vi "set_PSG.vi"(4 "PSG1 frequency":dbl) -> ()   [LabVIEW 2011]
doc: "sets PSG1 and PSG2 frequencies based on the frequency wired to the vi and the frequency offset stored in the global"
uses:
  global.vi
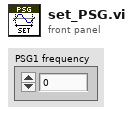
[diagram p1: front panel]
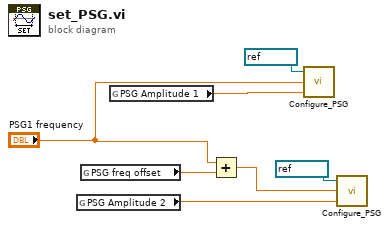
[diagram p0: block diagram]
diagram:
  n1 = global read "global.vi" "PSG Amplitude 2"() -> (w5:dbl)
  n2 = global read "global.vi" "PSG freq offset"() -> (w3:dbl)
  n3 = global read "global.vi" "PSG Amplitude 1"() -> (w4:dbl)
  n4 = Add(x="PSG1 frequency", y=w3) -> (x+y=w2:dbl)
  n5 = call "Configure_PSG.vi"("Power [dBm]"=w4, "Frequency [GHz]"="PSG1 frequency", "VISA resource name"=refnum<visa-resource-name> "PSG1") -> ()  [unwired: 2 in]
  n6 = call "Configure_PSG.vi"("Power [dBm]"=w5, "Frequency [GHz]"=w2, "VISA resource name"=refnum<visa-resource-name> "PSG2") -> ()  [unwired: 2 in]
